vi "readbin(logical).vi"(9 "Legnth":i32=8, 10 "Offset":i32, 11 "Buffer INÂ":string) -> (1 "Logical":bool, 2 "Offset+Length":i32, 3 "Buffer OUT":string)   [LabVIEW 2017, in "HEKAdat.lvclass"]
uses:
  HEKAdat.lvclass
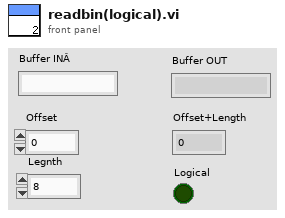
[diagram p1: front panel]
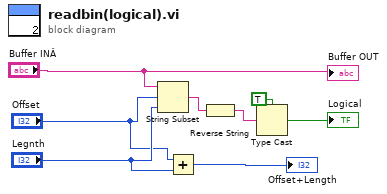
[diagram p0: block diagram]
diagram:
  n1 = String Subset(string="Buffer INÂ", offset (0)="Offset", length (rest)="Legnth") -> (substring=w3:string)
  n2 = Add(x="Offset", y="Legnth") -> (x+y=→"Offset+Length":i32)
  n3 = Reverse String(1:w3) -> (0:w4:string)
  n4 = Type Cast(type=TRUE, x=w4) -> (*(type *) &x=→"Logical":bool)
  "Buffer OUT" <- "Buffer INÂ"
